vi "test Import Export RAF CD.vi"(8 "error in (no error)":errorcluster, 11 "TestCase in":refnum<class "Routing and Faulting Scripting Unit Tests.lvclass">) -> (0 "error out":errorcluster, 3 "TestCase out":refnum<class "Routing and Faulting Scripting Unit Tests.lvclass">)   [LabVIEW 2017, in "Routing and Faulting Scripting Unit Tests.lvclass"]
uses:
  Routing and Faulting Scripting Unit Tests.lvclass
  Shared/Channel States.ctl
  Shared/Routing State.ctl
  Shared/Connection.ctl
  Routing and Faulting Scripting Unit Tests.lvclass/Routing and Faulting Scripting Unit Tests.ctl
  <userlib>/_OpenG.lib/file/file.llb/Append Path to Root if Relative - Scalar__ogtk.vi
  <vilib>/addons/_JKI Toolkits/VI Tester/TestCase.llb/TestCase.lvclass
  Routing and Faulting Scripting.lvlib
  Shared/Routing and Faulting Shared.lvlib
  niveristand-custom-device-testing-tools/VeriStandTestUtilities/VeriStandTestUtilities.lvlib
  C:/Program Files (x86)/National Instruments/LabVIEW 2017/vi.lib/addons/_JKI Toolkits/VI Tester/TestCase.llb/TestCase.lvclass
panel:
  in  "Save?":bool
  out "Output Filename":string
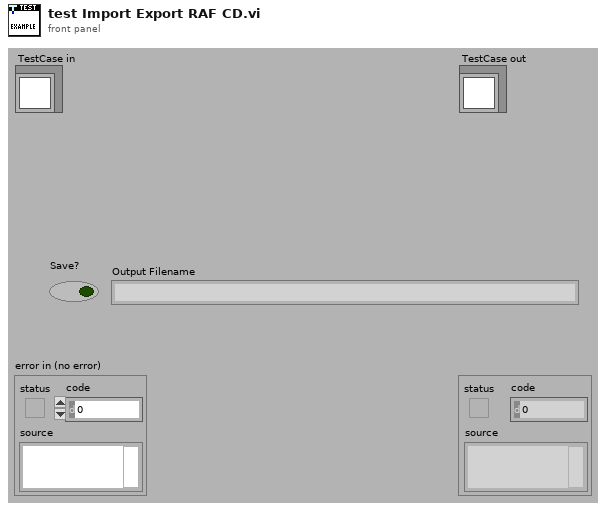
[diagram p1: front panel]
types:
  T1 = enum16{"open", "replace", "create", "open or create", "replace or create", "replace or create with confirmation"}
  T2 = typedef "Routing and Faulting Shared.lvlib/Channel States.ctl" = T3[]
  T3 = typedef "Routing and Faulting Shared.lvlib/Routing State.ctl" = cluster{"Name":string, "Description":string, "Value":i32, "Connection List":T4[]}
  T4 = typedef "Routing and Faulting Shared.lvlib/Connection.ctl" = cluster{"Module":string, "Source":string, "Destination":string}
  T5 = typedef "Custom Device API.lvlib/Custom Device Item Ref.ctl" = u64
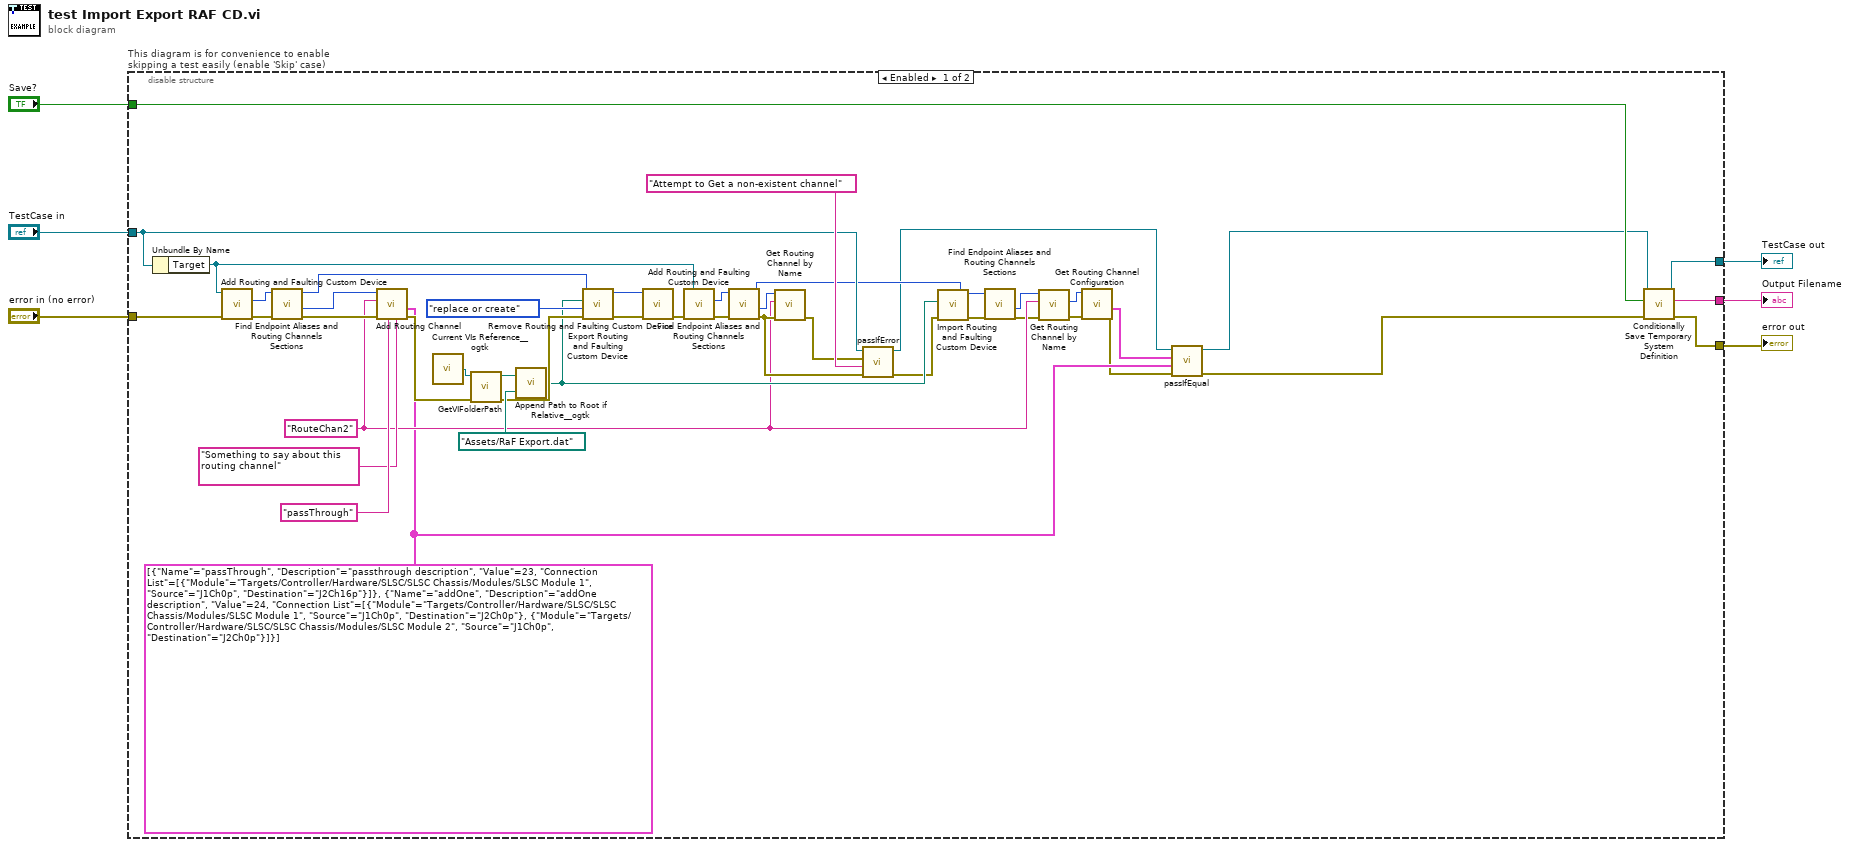
[diagram p0: block diagram]
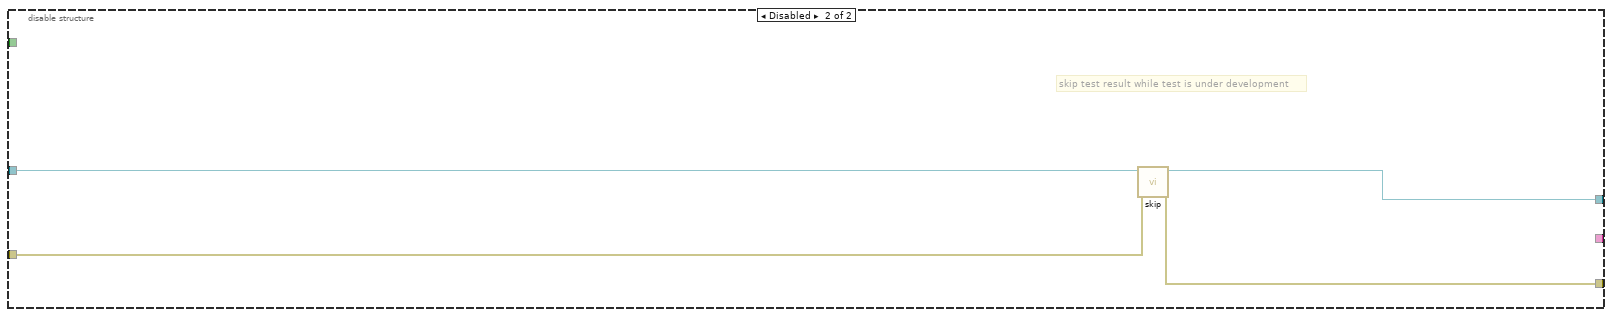
[diagram p2: hidden frame]
diagram:
  n1 = disable-structure "This diagram is for convenience to enable skipping a test easily (enable 'Skip' case)" shown="Enabled" {
    disable-tunnel: "TestCase in" -> [w31 w55]
    disable-tunnel: [w47 w53] -> w3
    disable-tunnel: [w50 w54] -> w5
    disable-tunnel: "error in (no error)" -> [w51 w52]
    disable-tunnel: [w49 _] -> w2
    disable-tunnel: "Save?" -> [w48 _]
    frame Enabled {
      w9 = T2 [{"Name"="passThrough", "Description"="passthrough description", "Value"=23, "Connection List"=[{"Module"="Targets/Controller/Hardware/SLSC/SLSC Chassis/Modules/SLSC Module 1", "Source"="J1Ch0p", "Destination"="J2Ch16p"}]}, {"Name"="addOne", "Description"="addOne description", "Value"=24, "Connection List"=[{"Module"="Targets/Controller/Hardware/SLSC/SLSC Chassis/Modules/SLSC Module 1", "Source"="J1Ch0p", "Destination"="J2Ch0p"}, {"Module"="Targets/Controller/Hardware/SLSC/SLSC Chassis/Modules/SLSC Module 2", "Source"="J1Ch0p", "Destination"="J2Ch0p"}]}] ("Channel States")
      w16 = "RouteChan2" ("Channel Name")
      n2 = Unbundle By Name(w31) -> ("Target"=w29:refnum<k24>)
      n3 = call "Add Routing and Faulting Custom Device.vi"("error in (no error)"=w51, "Target in"=w29) -> ("error out"=w46:errorcluster, "Routing and Faulting Custom Device Ref"=w44:T5)  [unwired: 7 in, 1 out]
      n4 = call "Find Endpoint Aliases and Routing Channels Sections.vi"("error in (no error)"=w46, "Routing and Faulting Custom Device Ref in"=w44) -> ("error out"=w41:errorcluster, "Routing Channels Ref"=w42:T5, "Routing and Faulting Custom Device Ref out"=w37:T5)  [unwired: 6 in, 1 out]
      n5 = call "Add Routing Channel.vi"("Description"="Something to say about this routing channel", "Initial State"="passThrough" ("Name"), "error in (no error)"=w41, "State Configurations"=w9, "Channel Name"=w16, "Routing Channels Ref in"=w42) -> ("error out"=w45:errorcluster)  [unwired: 3 in, 2 out]
      n6 = call <userlib>:"Current VIs Reference__ogtk.vi"() -> ("Current VI's reference"=w40:refnum<vi>)  [unwired: 5 in]
      n7 = call "GetVIFolderPath.vi"("error in (no error)"=w45, "VI Reference in"=w40) -> ("error out"=w36:errorcluster, "VI Folder Path out"=w39:path)  [unwired: 8 in]
      n8 = call-poly <userlib>:"Append Path to Root if Relative__ogtk.vi"("Absolute or Relative Path"=path "Assets/RaF Export.dat", "Root Path"=w39) -> ("Absolute or Appended Path"=w21:path)
      n9 = call "Export Routing and Faulting Custom Device.vi"("error in (no error)"=w36, "operation"=T1."replace or create", "Path"=w21, "Routing and Faulting Custom Device Ref in"=w37) -> ("error out"=w33:errorcluster, "Routing and Faulting Custom Device Ref out"=w34:T5)  [unwired: 6 in]
      n10 = call "Remove Routing and Faulting Custom Device.vi"("error in (no error)"=w33, "Routing and Faulting Custom Device Ref"=w34) -> ("error out"=w28:errorcluster)  [unwired: 9 in]
      n11 = call "Add Routing and Faulting Custom Device.vi"("error in (no error)"=w28, "Target in"=w29) -> ("error out"=w27:errorcluster, "Routing and Faulting Custom Device Ref"=w26:T5)  [unwired: 7 in, 1 out]
      n12 = call "Find Endpoint Aliases and Routing Channels Sections.vi"("error in (no error)"=w27, "Routing and Faulting Custom Device Ref in"=w26) -> ("error out"=w23:errorcluster, "Routing Channels Ref"=w25:T5, "Routing and Faulting Custom Device Ref out"=w22:T5)  [unwired: 6 in, 1 out]
      n13 = call "Get Routing Channel by Name.vi"("error in (no error)"=w23, "Channel Name"=w16, "Routing Channels Ref in"=w25) -> ("error out"=w24:errorcluster)  [unwired: 6 in, 2 out]
      n14 = call-dynamic "passIfError.vi"("error in (no error)"=w23, "task (\"\")"="Attempt to Get a non-existent channel" ("task (\"\")"), "error"=w24, "TestCase in"=w31) -> ("error out"=w20:errorcluster, "TestCase out"=w14:refnum<class "Routing and Faulting Scripting Unit Tests.lvclass">)  [unwired: 6 in]
      n15 = call "Import Routing and Faulting Custom Device.vi"("error in (no error)"=w20, "Path"=w21, "Routing and Faulting Custom Device Ref in"=w22) -> ("error out"=w19:errorcluster, "Routing and Faulting Custom Device Ref out"=w18:T5)  [unwired: 7 in]
      n16 = call "Find Endpoint Aliases and Routing Channels Sections.vi"("error in (no error)"=w19, "Routing and Faulting Custom Device Ref in"=w18) -> ("error out"=w15:errorcluster, "Routing Channels Ref"=w17:T5)  [unwired: 6 in, 2 out]
      n17 = call "Get Routing Channel by Name.vi"("error in (no error)"=w15, "Channel Name"=w16, "Routing Channels Ref in"=w17) -> ("error out"=w11:errorcluster, "Channel Ref"=w12:T5)  [unwired: 6 in, 1 out]
      n18 = call "Get Routing Channel Configuration.vi"("error in (no error)"=w11, "Channel Ref in"=w12) -> ("error out"=w8:errorcluster, "State Configurations"=w10:T2)  [unwired: 4 in, 4 out]
      n19 = call-dynamic "passIfEqual.vi"("error in (no error)"=w8, "y"=w9, "x"=w10, "TestCase in"=w14) -> ("error out"=w7:errorcluster, "TestCase out"=w13:refnum<class "Routing and Faulting Scripting Unit Tests.lvclass">)  [unwired: 6 in]
      n20 = call "Conditionally Save Temporary System Definition.vi"("error in (no error)"=w7, "Save?"=w48, "Test Case"=w13) -> ("error out"=w50:errorcluster, "filename"=w49:string, "Test Case"=w47:refnum<class "Routing and Faulting Scripting Unit Tests.lvclass">)  [unwired: 6 in]
    }
    frame Disabled {
      # "skip test result while test is under development"
      n21 = call <vilib>:"skip.vi"("error in (no error)"=w52, "TestCase in"=w55) -> ("error out"=w54:errorcluster, "TestCase out"=w53:refnum<class "Routing and Faulting Scripting Unit Tests.lvclass">)  [unwired: 8 in]
    }
  }
  "error out" <- w5
  "TestCase out" <- w3
  "Output Filename" <- w2
